vi "setEventId.vi"(8 "error in (no error)":errorcluster, 10 "eventId":dbl, 11 "RampEvent in":refnum<class "RampEvent.lvclass">) -> (0 "error out":errorcluster, 3 "RampEvent out":refnum<class "RampEvent.lvclass">)   [LabVIEW 2009, in "Tools.lvlib" / "Scripting.lvlib" / "RampEvent.lvclass"]
uses:
  RampEvent.lvclass
  ScriptEvent.lvclass
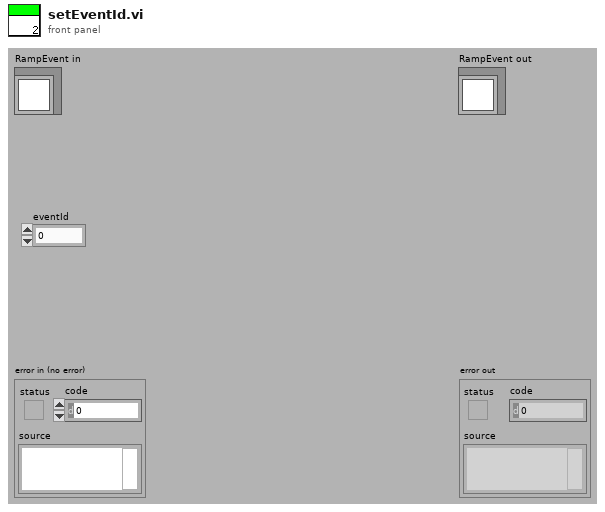
[diagram p1: front panel]
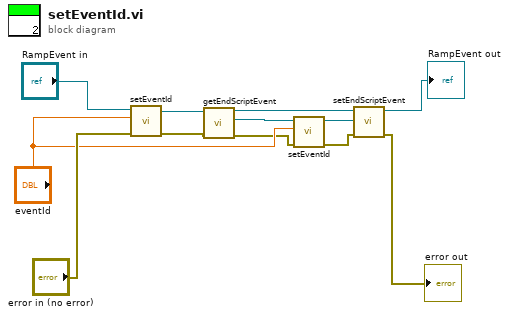
[diagram p0: block diagram]
diagram:
  n1 = call-parent "setEventId.vi"("error in (no error)"="error in (no error)", "eventId"="eventId", "ScriptEvent in"="RampEvent in") -> ("error out"=w6:errorcluster, "ScriptEvent out"=w10:refnum<class "RampEvent.lvclass">)  [unwired: 7 in]
  n2 = call "getEndScriptEvent.vi"("error in (no error)"=w6, "RampEvent.lvclass in"=w10) -> ("error out"=w7:errorcluster, "ScriptEvent.lvclass"=w9:refnum<class "ScriptEvent.lvclass">, "RampEvent.lvclass out"=w4:refnum<class "RampEvent.lvclass">)  [unwired: 7 in]
  n3 = call-parent "setEventId.vi"("error in (no error)"=w7, "eventId"="eventId", "ScriptEvent in"=w9) -> ("error out"=w3:errorcluster, "ScriptEvent out"=w5:refnum<class "ScriptEvent.lvclass">)  [unwired: 7 in]
  n4 = call "setEndScriptEvent.vi"("error in (no error)"=w3, "endScriptEvent.lvclass"=w5, "RampEvent.lvclass in"=w4) -> ("error out"=→"error out":errorcluster, "RampEvent.lvclass out"=→"RampEvent out":refnum<class "RampEvent.lvclass">)  [unwired: 7 in]
